vi "Initialise.vi"(8 "error in (no error)":errorcluster, 10 "System In":refnum<class "abs_System.lvclass">, 11 "Node in":refnum<class "abs_Type Leaf.lvclass">) -> (0 "error out":errorcluster, 2 "System Out":refnum<class "abs_System.lvclass">, 3 "Node out":refnum<class "abs_Type Leaf.lvclass">)   [LabVIEW 2021, in "BT.lvlib" / "abs_Type Leaf.lvclass"]
uses:
  abs_Type Leaf.lvclass
  abs_Leaf/abs_Leaf.lvclass
  GitHub/LV_Abstract/Source/Abs_Types/Type/Abs_Type.lvclass
  abs_System/abs_System.lvclass
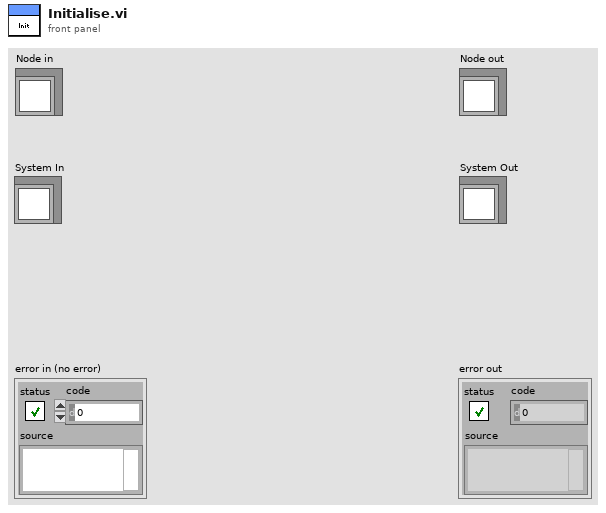
[diagram p1: front panel]
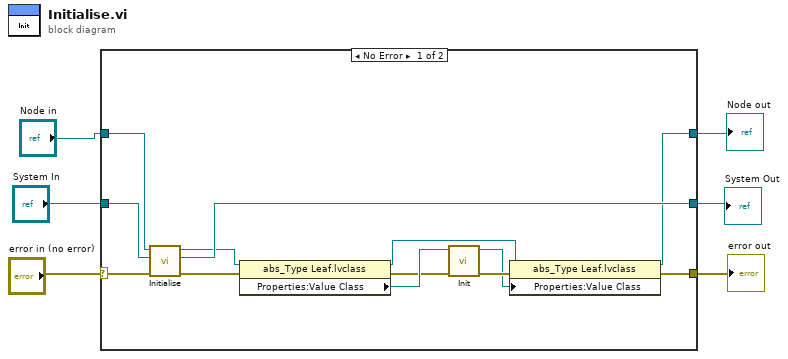
[diagram p0: block diagram]
diagram:
  n1 = case shown="No Error" "error in (no error)" {
    selector: "error in (no error)" -> [w18 w20]
    tunnel: [w19 w21] -> w3
    tunnel: "System In" -> [w17 w21]
    tunnel: "Node in" -> [w16 w22]
    tunnel: [w12 w20] -> w6
    tunnel: [w7 w22] -> w2
    frame No Error {
      n2 = call-parent "Initialise.vi"("error in (no error)"=w18, "System In"=w17, "Node in"=w16) -> ("error out"=w15:errorcluster, "System Out"=w19:refnum<class "abs_System.lvclass">, "Node out"=w14:refnum<class "abs_Type Leaf.lvclass">)  [unwired: 6 in]
      n3 = property class="abs_Type Leaf.lvclass"(reference=w14, error in=w15) -> (reference out=w13:refnum<class "abs_Type Leaf.lvclass">, error out=w10:errorcluster, "Properties:Value Class"=w11:refnum<class "Abs_Type.lvclass">)
      n4 = call-dynamic "Init.vi"("error in (no error)"=w10, "Data in"=w11) -> ("error out"=w9:errorcluster, "Data out"=w8:refnum<class "Abs_Type.lvclass">)  [unwired: 8 in]
      n5 = property class="abs_Type Leaf.lvclass"(reference=w13, error in=w9, "Properties:Value Class"=w8) -> (reference out=w7:refnum<class "abs_Type Leaf.lvclass">, error out=w12:errorcluster)
    }
    frame Error {
    }
  }
  "error out" <- w6
  "Node out" <- w2
  "System Out" <- w3
